vi "Compatibility Triggered Acquisition.vi"() -> ()   [LabVIEW 2023]
doc: "The Compatibility Triggered Acquisition example uses an external or RTSI trigger to trigger an image acquisition. This VI configures and acquires images based on the trigger parameters specified.\n\nThis example uses the IMAQdx driver to interface with a Camera Link frame grabber. It uses the NI-IMAQdx Compatibility for NI-IMAQ API to facilitate migration between the two drivers. The NI-IMAQdx VIs are drop-in replacements to existing NI-IMAQ VIs."
uses:
  <vilib>/vision/driver/IMAQdx.llb/IMAQdx Acquisition Mode.ctl
  <vilib>/vision/driver/IMAQdx.llb/IMAQdx Buffer Number Mode.ctl
  <vilib>/vision/driver/NI_Vision_Acquisition_Software.lvlib
panel:
  in  "Interface Name":refnum<k21> caption="IMAQdx Session"
  in  "Trigger Polarity":u32(ring) items=["Rising Edge", "Falling Edge"]
  in  "Frame Timeout (ms)":u32=1000
  in  "Trigger Line Number":u32
  in  "Trigger Type":u32(ring) items=["External"=0, "RTSI"=1, "ISO In"=2, "Scaled Encoder"=5]
  out "Frame Rate":dbl
  in  "Stop":bool
  out "Last Valid Buffer":u32
  out "Image":T1(plugin-control)
  # "Overview: Demonstrates how to configure a triggered ring acquisition based on the trigger settings.\nRequirements: Vision Acquisition Software 18.0 or later, PCIe-1427, PCIe-1433, PXIe-1435, or PCIe-1437 frame grabber.\nInstructions: \n1. Select the Camera Link frame grabber Interface Name.\n2. Run the VI.\n3. Drive the specified Trigger Line to the specified Polarity to trigger every image."
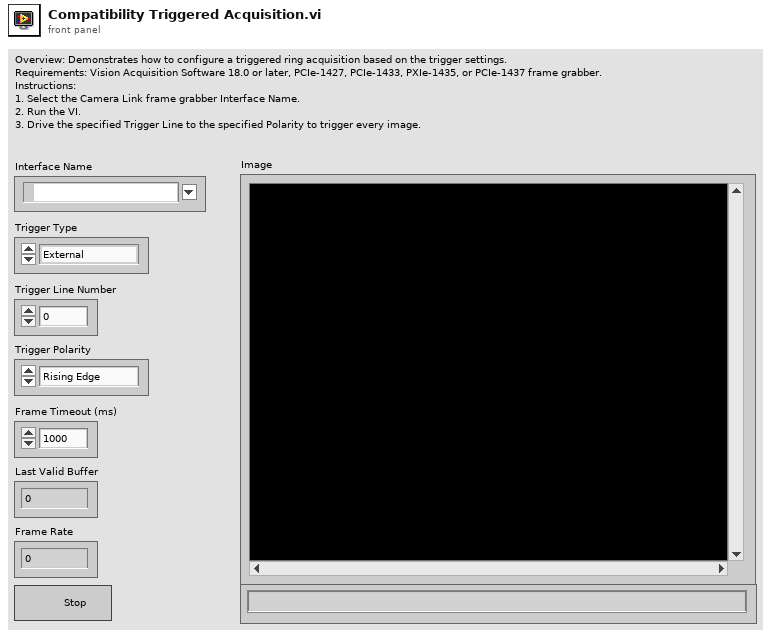
[diagram p1: front panel]
types:
  T1 = typedef "IMAQ Image.ctl" = refnum<image>
  T2 = typedef "NI_Vision_Acquisition_Software.lvlib/IMAQdx Acquisition Mode.ctl" = enum32{"One Shot", "Continuous"}
  T3 = typedef "IMAQdx.ctl" = refnum<k21>
  T4 = typedef "NI_Vision_Acquisition_Software.lvlib/IMAQdx Buffer Number Mode.ctl" = enum32{"Next", "Last", "Buffer Number", "Every", "Last New"}
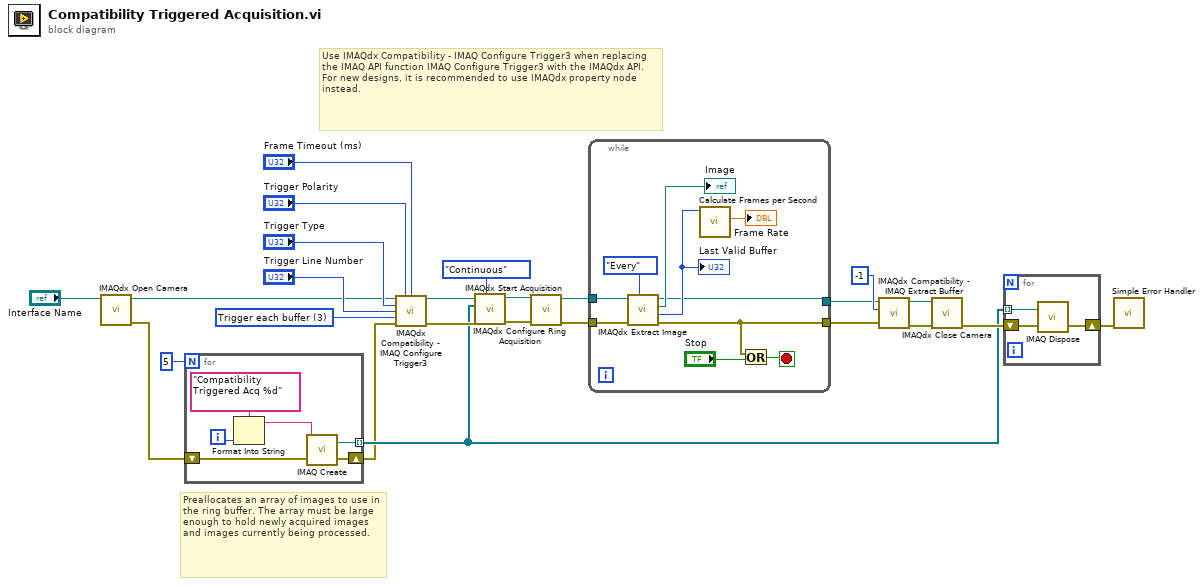
[diagram p0: block diagram]
diagram:
  w21 = u32 3 items=["Disabled", "Trigger start of acquisition", "Trigger start of each buffer list", "Trigger each buffer", "Trigger each line (linescan)", "Trigger end of acquisition"] ("Action")
  # "Use IMAQdx Compatibility - IMAQ Configure Trigger3 when replacing the IMAQ API function IMAQ Configure Trigger3 with the IMAQdx API. For new designs, it is recommended to use IMAQdx property node instead."
  # "Preallocates an array of images to use in the ring buffer. The array must be large enough to hold newly acquired images and images currently being processed."
  n1 = call <vilib>:"IMAQdx Open Camera.vi"("Session In"="Interface Name") -> ("error out"=w24:errorcluster, "Session Out"=w2:T3)  [unwired: 9 in]
  n2 = for {
    N: 5 -> [_]
    tunnel: [w30] -> w6 mode=indexing
    shift-right: [w29] -> w3
    shift-left: w24 -> [w31]
    i -> [w28]
    n3 = Format Into String(format string="Compatibility Triggered Acq %d" ("Image Name"), w28) -> (resulting string=w27:string)  [unwired: 2 in, 1 out]
    n4 = call "IMAQ Create"("Image Name"=w27, "error in (no error)"=w31) -> ("New Image"=w30:T1, "error out"=w29:errorcluster)  [unwired: 2 in, 1 out]
  }
  n5 = call <vilib>:"IMAQdx Compatibility - IMAQ Configure Trigger3.vi"("Session In"=w2, "Polarity"="Trigger Polarity", "Frame timeout (ms)"="Frame Timeout (ms)", "Type"="Trigger Type", "Line Number"="Trigger Line Number", "Action"=w21, "error in (no error)"=w3) -> ("Session Out"=w8:T3, "error out"=w7:errorcluster)  [unwired: 7 in]
  n6 = call <vilib>:"IMAQdx Configure Ring Acquisition.vi"("Mode"=IMAQdx_Acquisition_Mode."Continuous" ("Continuous?"), "error in"=w7, "Images"=w6, "Session In"=w8) -> ("error out"=w4:errorcluster, "Session Out"=w5:T3)  [unwired: 5 in, 1 out]
  n7 = call <vilib>:"IMAQdx Start Acquisition.vi"("error in"=w4, "Session In"=w5) -> ("error out"=w17:errorcluster, "Session Out"=w18:T3)  [unwired: 8 in]
  n8 = while {
    tunnel: w18 -> [w41]
    tunnel: w17 -> [w40]
    tunnel: [w36] -> w15
    tunnel: [w33] -> w12
    stop <- w34 stop-if-true
    n9 = call <vilib>:"IMAQdx Extract Image.vi"("Buffer Number Mode (Next)"=IMAQdx_Buffer_Number_Mode."Every", "error in"=w40, "Session In"=w41) -> ("error out"=w36:errorcluster, "Buffer Number Out"=w38:u32, "Image Out"=→"Image":T1, "Session Out"=w33:T3)  [unwired: 5 in]
    "Last Valid Buffer" <- w38
    n10 = call <vilib>:"Calculate Frames per Second.vi"("Buffer Number"=w38) -> ("Processed Frames/s"=→"Frame Rate":dbl)  [unwired: 8 in, 2 out]
    n11 = Or(x=w36, y="Stop") -> (x .or. y?=w34:bool)
  }
  n12 = call <vilib>:"IMAQdx Compatibility - IMAQ Extract Buffer.vi"("error in (no error)"=w15, "Buffer to extract"=-1, "Session In"=w12) -> ("error out"=w14:errorcluster, "Session Out"=w11:T3)  [unwired: 3 in, 4 out]
  n13 = call <vilib>:"IMAQdx Close Camera.vi"("error in"=w14, "Session In"=w11) -> ("error out"=w9:errorcluster)  [unwired: 9 in]
  n14 = for {
    shift-right: [w43] -> w10
    shift-left: w9 -> [w44]
    tunnel: w6 -> [w42] mode=indexing
    n15 = call "IMAQ Dispose"("Image"=w42, "error in (no error)"=w44) -> ("error out"=w43:errorcluster)  [unwired: 4 in]
  }
  n16 = call <vilib>:"Simple Error Handler.vi"("error in (no error)"=w10) -> ()  [unwired: 4 in, 5 out]
